vi "Run Action.vi"(8 "error in":errorcluster, 11 "Action In":refnum<class "Auton Action Base.lvclass">) -> (0 "error out":errorcluster)   [LabVIEW 2016, in "Auton Mode Base.lvclass"]
uses:
  Auton Mode Base.lvclass
  Actions/Actions Base/Auton Action Base.lvclass
  Private/Auton Abort Global.vi
  Private/Call Action Dynamic.vi
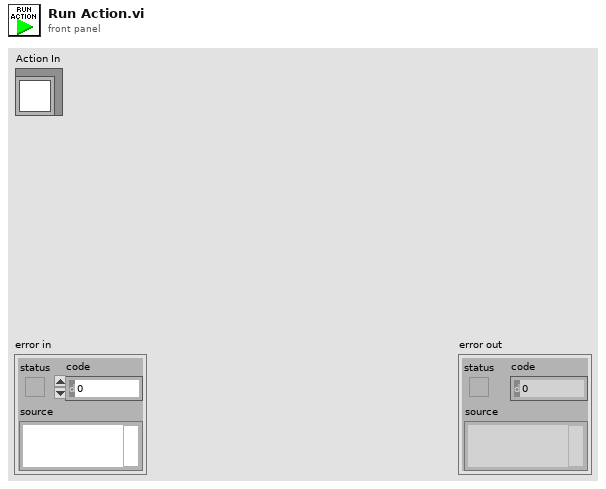
[diagram p1: front panel]
types:
  T1 = typedef "Auton Mode Base.lvclass/Auton Action Monitor Type.ctl" = cluster{"Min Voltage (V)":dbl, "PDP Fault?":bool, "Run Time ms":u32, "Max Currents (A)":dbl[]}
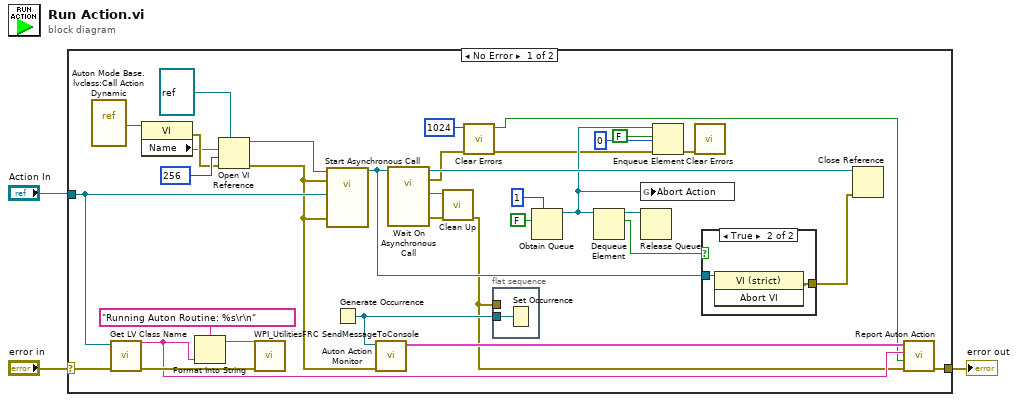
[diagram p0: block diagram]
diagram:
  n1 = case shown="No Error" "error in" {
    selector: "error in" -> [w34 w41]
    tunnel: [w35 w41] -> w2
    tunnel: "Action In" -> [w23 _]
    frame No Error {
      n2 = vi-ref "Auton Mode Base.lvclass:Call Action Dynamic.vi"() -> (w26:refnum<vi>)
      n3 = call <vilib>:"Get LV Class Name.vi"("error in (no error)"=w34, "object"=w23) -> ("error out"=w33:errorcluster, "class name"=w30:string)  [unwired: 8 in]
      n4 = property class="VI"(reference=w26) -> (error out=w25:errorcluster, "Name"=w24:string)  [unwired: 1 in, 1 out]
      n5 = Format Into String(format string="Running Auton Routine: %s\r\n", w30) -> (resulting string=w32:string)  [unwired: 2 in, 1 out]
      n6 = Open VI Reference(type specifier VI Refnum (for type only)=refnum<vi> refnum, vi path=w24, options=256, error in (no error)=w25) -> (vi reference=w29:refnum<vi>, error out=w22:errorcluster)  [unwired: 1 in, 1 out]
      n7 = call <vilib>:"WPI_UtilitiesFRC SendMessageToConsole.vi"("Message"=w32, "error in (no error)"=w33) -> ()  [unwired: 13 in, 1 out]
      n8 = call-by-ref "Start Asynchronous Call"(reference=w29, error in=w22, 8:"error in (no error)"=w22, "Auton Action Base in"=w23) -> (reference out=w15:refnum<vi>)  [unwired: 8 in, 3 out]
      n9 = Generate Occurrence() -> (w37:refnum<k4>)
      n10 = call "Auton Action Monitor.vi"("error in"=w22, "occurrence"=w37) -> ("Auton Monitor"=w36:T1)  [unwired: 8 in, 1 out]
      n11 = call-by-ref "Wait On Asynchronous Call"(reference=w15) -> (reference out=w21:refnum<vi>, error out=w10:errorcluster, 0:"error out"=w6:errorcluster, "Auton Action Base out"=w14:refnum<class "Auton Action Base.lvclass">)  [unwired: 11 in]
      n12 = call-dynamic "Clean Up.vi"("error in (no error)"=w6, "Auton Action Base in"=w14) -> ("error out"=w5:errorcluster)  [unwired: 8 in, 1 out]
      n13 = call <vilib>:"Clear Errors.vi"("error in (no error)"=w10, "specific error code to clear (0: all)"=1024) -> ("error out"=w9:errorcluster, "specific error cleared?"=w7:bool)  [unwired: 4 in]
      n14 = flat-sequence {
        tunnel: w37 -> [w40]
        tunnel: w5 -> [_]
        frame #0 {
          n15 = Set Occurrence(w40) -> ()
        }
      }
      n16 = Obtain Queue(max queue size (-1, unlimited)=1, element data type=FALSE) -> (queue out=w13:refnum<queue>)  [unwired: 3 in, 2 out]
      n17 = Dequeue Element(queue=w13) -> (queue out=w17:refnum<queue>, element=w18:bool)  [unwired: 2 in, 2 out]
      n18 = global write "Auton Abort Global.vi" "Abort Action"(w13) -> ()
      n19 = Release Queue(queue=w17) -> ()  [unwired: 2 in, 3 out]
      n20 = Enqueue Element(queue=w13, element=FALSE, timeout in ms (-1)=0, error in (no error)=w9) -> (error out=w11:errorcluster)  [unwired: 2 out]
      n21 = call <vilib>:"Clear Errors.vi"("error in (no error)"=w11) -> ()  [unwired: 5 in, 2 out]
      n22 = case shown="True" w18 {
        tunnel: [_ w39] -> w20
        tunnel: w15 -> [_ w38]
        frame False {
        }
        frame True {
          n23 = invoke class="VI (strict)" method="Abort VI"(reference=w38) -> (error out=w39:errorcluster)  [unwired: 2 in, 2 out]
        }
      }
      n24 = Close Reference(reference=w21, error in (no error)=w20) -> ()  [unwired: 1 out]
      n25 = call "Report Auton Action.vi"("error in"=w5, "Aborted?"=w7, "Name"=w30, "Auton Monitor"=w36) -> ("error out"=w35:errorcluster)  [unwired: 7 in]
    }
    frame Error {
    }
  }
  "error out" <- w2
